vi "SubVI_CurrentSettings.vi"() -> (3 "Curr set val":dbl[](array[numeric]))   [LabVIEW 2016]
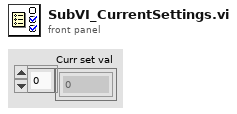
[diagram p1: front panel]
types:
  T1 = cluster{"Test Information":cluster{"date":string, "custom":string, "oper":string, "package":string, "pkg side":string, "solder":string, "brd side":string, "paste":string, "reflow":string}, "Sensor Set":cluster{"Accelerometer":cluster{"Sensitivity(mV/g)":dbl}, "Strain Guage":cluster{"Ch.":dbl[], "Gage factor":dbl[], "Resistance":dbl[], "Poisson ratio":dbl[]}}, "Resistor Set":cluster{"Criterion Level":dbl, "Res. Set":cluster{"Res. Ch":dbl, "Res. Active":bool, "Res Initial":dbl}[]}, "Test Stop Condition":cluster{"Test cycle":u16, "Fail number in a cycle":u16, "Fail factor":cluster{"Duration":u16, "Fail No.":u16}}, "Acceleration Condition ":cluster{"Shock duration pecent [%]":u16, "Filter cutoff freq":u32}, "Save":cluster{"Save Path":path, "File Name":string}}
  T2 = cluster{"Res. Ch":dbl, "Res. Active":bool, "Res Initial":dbl}[]
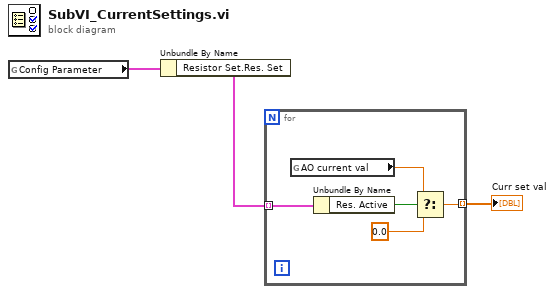
[diagram p0: block diagram]
diagram:
  n1 = global read "글로벌_Config Parameter.vi" "Config Parameter"() -> (w2:T1)
  n2 = Unbundle By Name(w2) -> ("Resistor Set.Res. Set"=w3:T2)
  n3 = for {
    tunnel: w3 -> [w8] mode=indexing
    tunnel: [w6] -> w1 mode=indexing
    n4 = global read "글로벌_Config Parameter.vi" "AO current val"() -> (w5:dbl)
    n5 = Unbundle By Name(w8) -> ("Res. Active"=w7:bool)
    n6 = Select(t=w5, s=w7, f=0.0) -> (s? t:f=w6:dbl)
  }
  "Curr set val" <- w1
